vi "Object Factory.vi"(6 "Ring Images In":variant, 8 "error in (no error)":errorcluster, 9 "Panel Origin":T1, 11 "GOject In":refnum<vi>) -> (0 "error out":errorcluster, 1 "Is Visible":bool, 2 "Is Control":bool, 3 "Object Out":refnum<class "Object.lvclass">, 4 "Ring Images Out":variant, 5 "Is Indicator":bool)   [LabVIEW 2015, in "Front Panel Publisher.lvlib" / "Web Front Panel.lvclass"]
doc: "Convert FP refs into \"HTML\" objects"
uses:
  Web Front Panel.lvclass
  Front Panel Objects/Object_class/Object.lvclass
  <vilib>/Utility/miscctls.llb/LVPointTypeDef.ctl
  Front Panel Objects/Object_class/Attributes.ctl
  Front Panel Objects/Object_class/Coordinates.ctl
  Front Panel Objects/Control_class/Attributes.ctl
  Front Panel Objects/Text_class/Text.lvclass
  Front Panel Objects/Boolean_class/Attributes.ctl
  Front Panel Objects/Numeric_class/Attributes.ctl
  Front Panel Objects/String_class/Attributes.ctl
  Front Panel Objects/Graph_class/Attributes.ctl
  Front Panel Objects/Select_class/Attributes.ctl
  Front Panel Objects/Progressbar_class/Attributes.ctl
  Front Panel Objects/Text_class/Attributes.ctl
  Front Panel Objects/Control_class/Control.lvclass
  Front Panel Objects/Boolean_class/Boolean.lvclass
  Front Panel Objects/Graph_class/Graph.lvclass
  Front Panel Objects/Numeric_class/Numeric.lvclass
  Front Panel Publisher.lvlib
  Front Panel Objects/String_class/String.lvclass
  Front Panel Objects/Select_class/Select.lvclass
  Front Panel Objects/Progressbar_class/Progressbar.lvclass
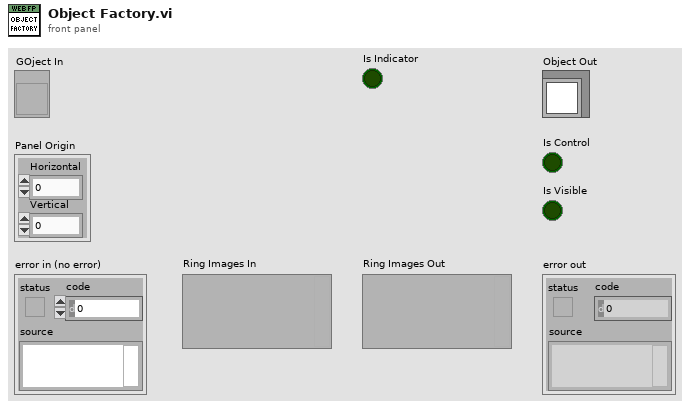
[diagram p1: front panel]
types:
  T1 = typedef "LVPointTypeDef.ctl" = cluster{"Horizontal":i16, "Vertical":i16}
  T2 = typedef "Front Panel Publisher.lvlib/Object.lvclass/Attributes.ctl" = cluster{"UID":i32, "Type":string, "Coordinates":T3, "Reference":refnum<vi>}
  T3 = typedef "Front Panel Publisher.lvlib/Object.lvclass/Coordinates.ctl" = cluster{"Left":i32, "Top":i32, "Height":u32, "Width":u32}
  T4 = typedef "Front Panel Publisher.lvlib/Control.lvclass/Attributes.ctl" = cluster{"Description":string, "Indicator":bool, "Default Value":variant, "Control Index":i32, "Label":refnum<class "Text.lvclass">, "Caption":refnum<class "Text.lvclass">, "Image b64":string, "Use Picture":bool, "Value Only":bool}
  T5 = typedef "Front Panel Publisher.lvlib/Boolean.lvclass/Attributes.ctl" = cluster{"Boolean ref":refnum<vi>, "Switching":bool, "Boolean Strings":string[], "Text":refnum<class "Text.lvclass">, "Images b64":string[]}
  T6 = typedef "Front Panel Publisher.lvlib/Numeric.lvclass/Attributes.ctl" = cluster{"unused":dbl}
  T7 = typedef "Front Panel Publisher.lvlib/String.lvclass/Attributes.ctl" = cluster{"unused":string}
  T8 = typedef "Front Panel Publisher.lvlib/Graph.lvclass/Attributes.ctl" = cluster{"X Label Text":string, "X Format String":string, "Y Label Text":string[], "Y Format String":string[], "Plot Y Axis Selection":enum16{"Y Axis", "Y2 Axis"}[], "Width":u32, "Series JSON Data":string}
  T9 = typedef "Front Panel Publisher.lvlib/Select.lvclass/Attributes.ctl" = cluster{"Ring Image Variable Name":string}
  T10 = typedef "Front Panel Publisher.lvlib/Progressbar.lvclass/Attributes.ctl" = cluster{"Maximum":dbl, "Minimum":dbl}
  T11 = cluster{"Object":T2, "Control":T4, "Boolean":T5, "Numeric":T6, "String":T7, "Graph":T8, "Select":T9, "Progressbar":T10, "Object out":refnum<class "Object.lvclass">, "Label":refnum<class "Text.lvclass">, "Caption":refnum<class "Text.lvclass">, "Is Indicator":bool, "Is Control":bool, "Is Visible":bool, "Ring Images":variant}
  T12 = typedef "Front Panel Publisher.lvlib/Text.lvclass/Attributes.ctl" = cluster{"Text":string, "Font":string, "Font Size":u32, "Visible":bool, "Control Reference":refnum<vi>}
  T13 = typedef "LVRectTypeDef.ctl" = cluster{"Left":i16, "Top":i16, "Right":i16, "Bottom":i16}
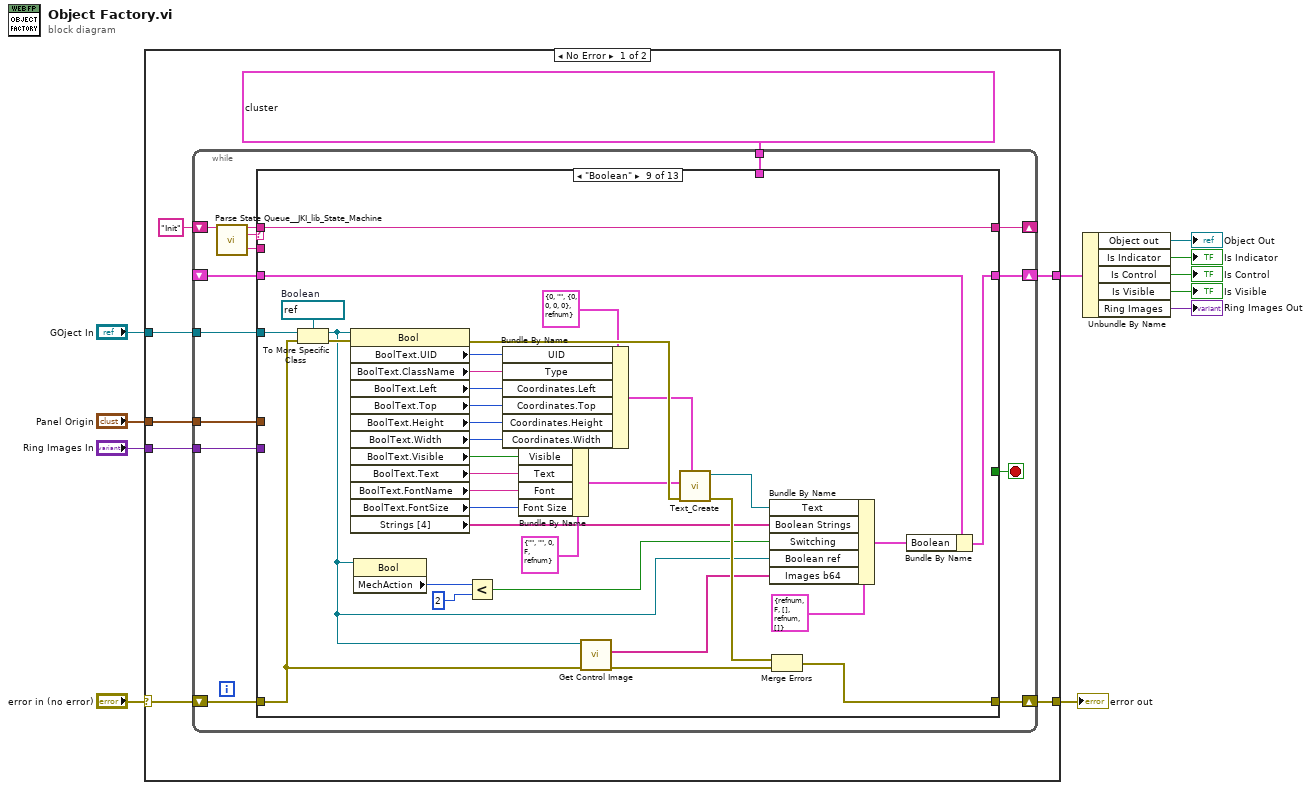
[diagram p0: block diagram]
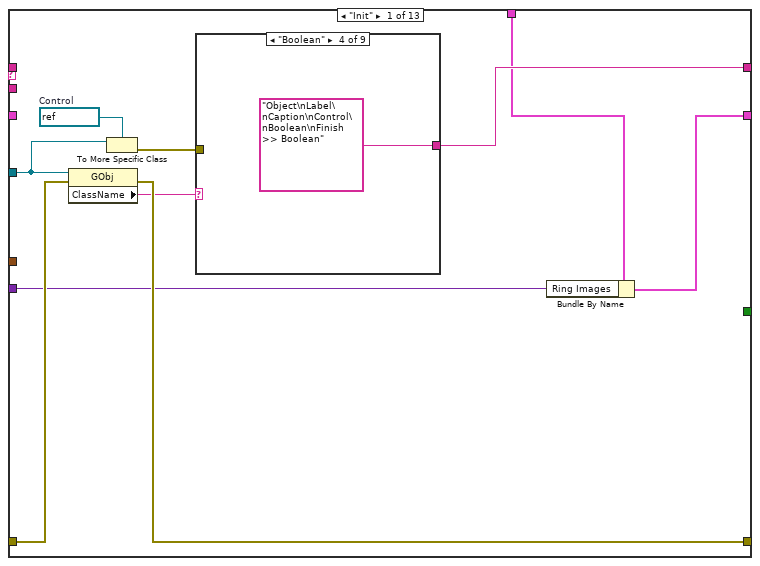
[diagram p2: hidden frame]
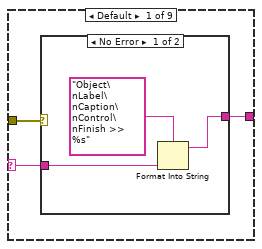
[diagram p3: hidden frame]
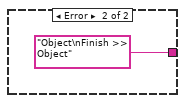
[diagram p4: hidden frame]
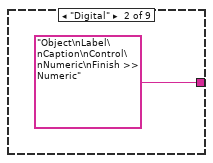
[diagram p5: hidden frame]
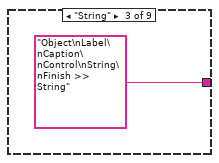
[diagram p6: hidden frame]
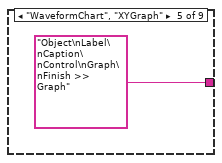
[diagram p7: hidden frame]
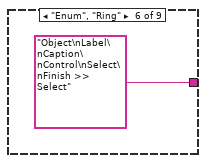
[diagram p8: hidden frame]
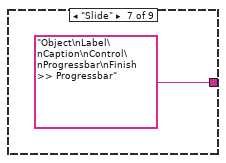
[diagram p9: hidden frame]
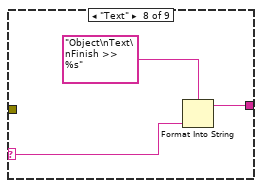
[diagram p10: hidden frame]
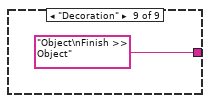
[diagram p11: hidden frame]
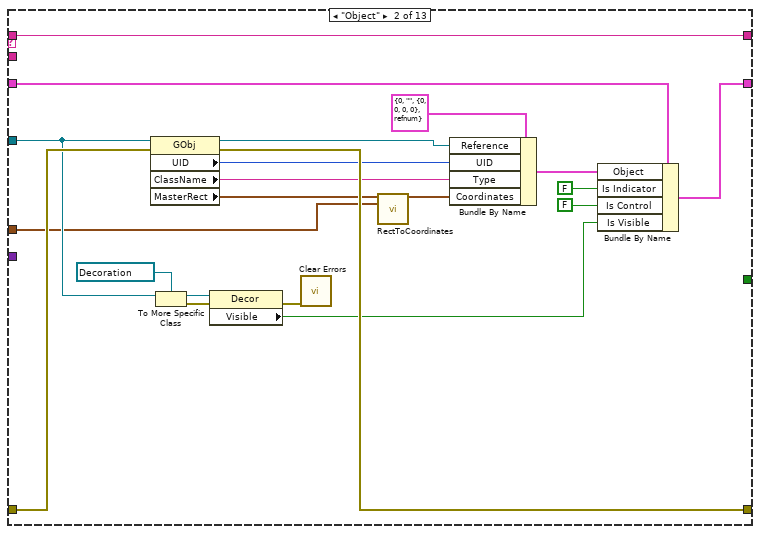
[diagram p12: hidden frame]
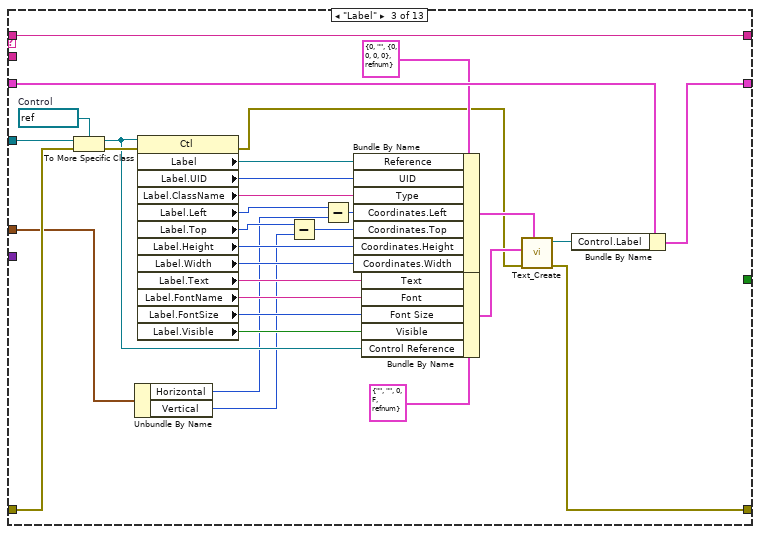
[diagram p13: hidden frame]
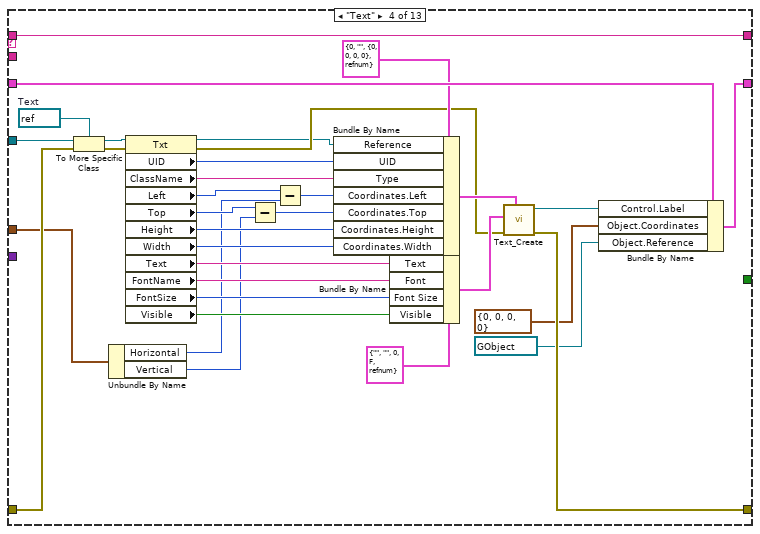
[diagram p14: hidden frame]
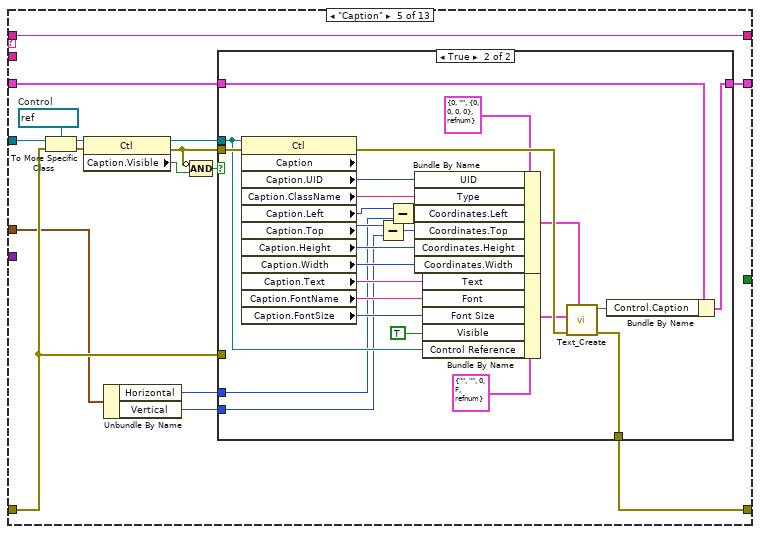
[diagram p15: hidden frame]
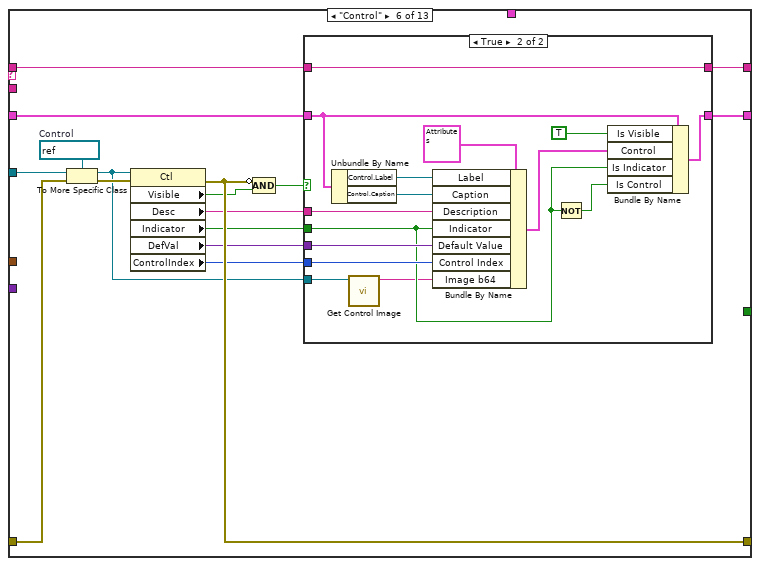
[diagram p17: hidden frame]
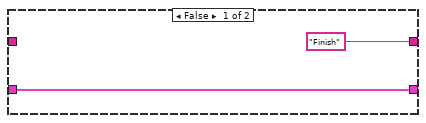
[diagram p18: hidden frame]
diagram:
  n1 = case shown="No Error" "error in (no error)" {
    selector: "error in (no error)" -> [w18 w353]
    tunnel: [w19 w353] -> w10
    tunnel: "GOject In" -> [w17 _]
    tunnel: [w14 _] -> w8
    tunnel: "Ring Images In" -> [w13 _]
    tunnel: "Panel Origin" -> [w12 _]
    frame No Error {
      n2 = while {
        tunnel: w17 -> [w31]
        shift-right: [w22] -> _
        shift-left: "Init" -> [w26]
        shift-right: [w30] -> w14
        shift-left: _ -> [w29]
        shift-right: [w32] -> w19
        shift-left: w18 -> [w33]
        tunnel: T11 {"Object"={"UID"=0, "Type"="", "Coordinates"={"Left"=0, "Top"=0, "Height"=0, "Width"=0}, "Reference"=refnum}, "Control"={"Description"="", "Indicator"=FALSE, "Default Value"=variant, "Control Index"=0, "Label"=refnum, "Caption"=refnum, "Image b64"="", "Use Picture"=FALSE, "Value Only"=FALSE}, "Boolean"={"Boolean ref"=refnum, "Switching"=FALSE, "Boolean Strings"=[], "Text"=refnum, "Images b64"=[]}, "Numeric"={"unused"=0.0}, "String"={"unused"=""}, "Graph"={"X Label Text"="", "X Format String"="", "Y Label Text"=[], "Y Format String"=[], "Plot Y Axis Selection"=[], "Width"=0, "Series JSON Data"=""}, "Select"={"Ring Image Variable Name"=""}, "Progressbar"={"Maximum"=0.0, "Minimum"=0.0}, "Object out"=refnum, "Label"=refnum, "Caption"=refnum, "Is Indicator"=FALSE, "Is Control"=FALSE, "Is Visible"=FALSE, "Ring Images"=variant} -> [w28]
        tunnel: w13 -> [w21]
        tunnel: w12 -> [w20]
        stop <- w27 stop-if-true
        n3 = call <vilib>:"Parse State Queue__JKI_lib_State_Machine.vi"("State Queue"=w26) -> ("Remaining States"=w23:string, "Current State"=w25:string, "Arguments"=w24:string)  [unwired: 12 in]
        n4 = case shown="\"Boolean\"" w25 {
          tunnel: w31 -> [w38 w68 w108 w141 w155 w200 _ _ w259 w267 w272 w285 _]
          tunnel: [w40 w75 w96 w129 w150 w191 w224 w227 w256 w271 w280 w291 ""] -> w22
          tunnel: [w35 w77 w97 w130 w151 w194 w223 w226 w257 w269 w278 w290 w293] -> w30
          tunnel: w29 -> [_ w76 w98 w131 w152 w199 w223 w226 w258 w270 w279 w289 w292]
          tunnel: [w42 w80 w110 w143 w159 w202 w222 w225 w229 w262 w276 w281 w297] -> w32
          tunnel: w33 -> [w43 w81 w111 w144 w158 w203 w222 w225 w230 w263 w273 w282 w297]
          tunnel: w28 -> [w39 _ _ _ _ _ _ _ _ _ _ _ _]
          tunnel: [_ _ _ _ _ _ _ _ _ _ _ _ TRUE] -> w27
          tunnel: w24 -> [_ _ _ _ _ _ _ _ _ _ _ _ w294]
          tunnel: w23 -> [_ w75 w96 w129 w150 w190 w224 w227 w256 w271 w280 w291 _]
          tunnel: w21 -> [w34 _ _ _ _ _ _ _ _ _ w275 _ _]
          tunnel: w20 -> [_ w61 w84 w115 w148 _ _ _ _ _ _ _ _]
          frame "Init" {
            w37 = refnum<vi> refnum  # Control
            n5 = property class="GObj"(reference=w38, error in=w43) -> (error out=w42:errorcluster, "ClassName"=w41:string)  [unwired: 1 out]
            n6 = To More Specific Class(target class=w37, reference=w38) -> (error out=w36:errorcluster)  [unwired: 1 in, 1 out]
            n7 = case shown="\"Boolean\"" w41 {
              selector: w41 -> [w44 _ _ _ _ _ _ w58 _]
              tunnel: [w46 "Object\nLabel\nCaption\nControl\nNumeric\nFinish >> Numeric" "Object\nLabel\nCaption\nControl\nString\nFinish >> String" "Object\nLabel\nCaption\nControl\nBoolean\nFinish >> Boolean" "Object\nLabel\nCaption\nControl\nGraph\nFinish >> Graph" "Object\nLabel\nCaption\nControl\nSelect\nFinish >> Select" "Object\nLabel\nCaption\nControl\nProgressbar\nFinish >> Progressbar" w57 "Object\nFinish >> Object"] -> w40
              tunnel: w36 -> [w45 _ _ _ _ _ _ _ _]
              frame Default {
                n8 = case shown="No Error" w45 {
                  tunnel: [w47 "Object\nFinish >> Object"] -> w46
                  tunnel: w44 -> [w49 _]
                  frame No Error {
                    n9 = Format Into String(format string="Object\nLabel\nCaption\nControl\nFinish >> %s", w49) -> (resulting string=w47:string)  [unwired: 2 in, 1 out]
                  }
                  frame Error {
                  }
                }
              }
              frame "Digital" {
              }
              frame "String" {
              }
              frame "Boolean" {
              }
              frame "WaveformChart", "XYGraph" {
              }
              frame "Enum", "Ring" {
              }
              frame "Slide" {
              }
              frame "Text" {
                n10 = Format Into String(format string="Object\nText\nFinish >> %s", w58) -> (resulting string=w57:string)  [unwired: 2 in, 1 out]
              }
              frame "Decoration" {
              }
            }
            n11 = Bundle By Name(cluster=w39, "Ring Images"=w34) -> (w35:T11)
          }
          frame "Object" {
            n12 = property class="GObj"(reference=w68, error in=w81) -> (reference out=w71:refnum<vi>, error out=w80:errorcluster, "UID"=w78:i32, "ClassName"=w79:string, "MasterRect"=w72:T13)
            n13 = To More Specific Class(target class=refnum<vi> refnum ("GOject"), reference=w68) -> (specific class reference=w67:refnum<vi>, error out=w66:errorcluster)  [unwired: 1 in]
            n14 = property class="Decor"(reference=w67, error in=w66) -> (error out=w65:errorcluster, "Visible"=w64:bool)  [unwired: 1 out]
            n15 = call <vilib>:"Clear Errors.vi"("error in (no error)"=w65) -> ()  [unwired: 5 in, 2 out]
            n16 = call "RectToCoordinates.vi"("Rect"=w72, "Panel Origin"=w61) -> ("Coordinates"=w70:T3)  [unwired: 13 in]
            n17 = Bundle By Name(cluster=T2 {"UID"=0, "Type"="", "Coordinates"={"Left"=0, "Top"=0, "Height"=0, "Width"=0}, "Reference"=refnum} ("Object Attributes"), "Reference"=w71, "UID"=w78, "Type"=w79, "Coordinates"=w70) -> (w73:T2)
            n18 = Bundle By Name(cluster=w76, "Object"=w73, "Is Indicator"=FALSE, "Is Control"=FALSE, "Is Visible"=w64) -> (w77:T11)
          }
          frame "Label" {
            w109 = refnum<vi> refnum  # Control
            n19 = To More Specific Class(target class=w109, reference=w108, error in=w111) -> (specific class reference=w87:refnum<vi>, error out=w112:errorcluster)
            n20 = Unbundle By Name(w84) -> ("Horizontal"=w83:i16, "Vertical"=w82:i16)
            n21 = property class="Ctl"(reference=w87, error in=w112) -> (error out=w90:errorcluster, "Label"=w88:refnum<vi>, "Label.UID"=w107:i32, "Label.ClassName"=w106:string, "Label.Left"=w105:i32, "Label.Top"=w104:i32, "Label.Height"=w103:u32, "Label.Width"=w102:u32, "Label.Text"=w101:string, "Label.FontName"=w100:string, "Label.FontSize"=w99:u32, "Label.Visible"=w89:bool)  [unwired: 1 out]
            n22 = Subtract(x=w104, y=w82) -> (x-y=w85:i32)
            n23 = Subtract(x=w105, y=w83) -> (x-y=w86:i32)
            n24 = Bundle By Name(cluster=T2 {"UID"=0, "Type"="", "Coordinates"={"Left"=0, "Top"=0, "Height"=0, "Width"=0}, "Reference"=refnum} ("Object Attributes"), "Reference"=w88, "UID"=w107, "Type"=w106, "Coordinates.Left"=w86, "Coordinates.Top"=w85, "Coordinates.Height"=w103, "Coordinates.Width"=w102) -> (w93:T2)
            n25 = Bundle By Name(cluster=T12 {"Text"="", "Font"="", "Font Size"=0, "Visible"=FALSE, "Control Reference"=refnum} ("Text Attributes"), "Text"=w101, "Font"=w100, "Font Size"=w99, "Visible"=w89, "Control Reference"=w87) -> (w92:T12)
            n26 = call "Text_Create.vi"("Object Attributes"=w93, "error in (no error)"=w90, "Text Attributes"=w92) -> ("error out"=w110:errorcluster, "Text Out"=w91:refnum<class "Text.lvclass">)  [unwired: 7 in]
            n27 = Bundle By Name(cluster=w98, "Control.Label"=w91) -> (w97:T11)
          }
          frame "Text" {
            w142 = refnum<vi> refnum  # Text
            n28 = To More Specific Class(target class=w142, reference=w141, error in=w144) -> (specific class reference=w121:refnum<vi>, error out=w145:errorcluster)
            n29 = Unbundle By Name(w115) -> ("Horizontal"=w114:i16, "Vertical"=w113:i16)
            n30 = property class="Txt"(reference=w121, error in=w145) -> (reference out=w120:refnum<vi>, error out=w123:errorcluster, "UID"=w140:i32, "ClassName"=w139:string, "Left"=w138:i32, "Top"=w137:i32, "Height"=w136:u32, "Width"=w135:u32, "Text"=w134:string, "FontName"=w133:string, "FontSize"=w132:u32, "Visible"=w122:bool)
            n31 = Subtract(x=w137, y=w113) -> (x-y=w116:i32)
            n32 = Subtract(x=w138, y=w114) -> (x-y=w117:i32)
            n33 = Bundle By Name(cluster=T2 {"UID"=0, "Type"="", "Coordinates"={"Left"=0, "Top"=0, "Height"=0, "Width"=0}, "Reference"=refnum} ("Object Attributes"), "Reference"=w120, "UID"=w140, "Type"=w139, "Coordinates.Left"=w117, "Coordinates.Top"=w116, "Coordinates.Height"=w136, "Coordinates.Width"=w135) -> (w126:T2)
            n34 = Bundle By Name(cluster=T12 {"Text"="", "Font"="", "Font Size"=0, "Visible"=FALSE, "Control Reference"=refnum} ("Text Attributes"), "Text"=w134, "Font"=w133, "Font Size"=w132, "Visible"=w122) -> (w125:T12)
            n35 = call "Text_Create.vi"("Object Attributes"=w126, "error in (no error)"=w123, "Text Attributes"=w125) -> ("error out"=w143:errorcluster, "Text Out"=w124:refnum<class "Text.lvclass">)  [unwired: 7 in]
            n36 = Bundle By Name(cluster=w131, "Control.Label"=w124, "Object.Coordinates"=T3 {"Left"=0, "Top"=0, "Height"=0, "Width"=0}, "Object.Reference"=refnum<vi> refnum) -> (w130:T11)
          }
          frame "Caption" {
            w157 = refnum<vi> refnum  # Control
            n37 = To More Specific Class(target class=w157, reference=w155, error in=w158) -> (specific class reference=w156:refnum<vi>, error out=w161:errorcluster)
            n38 = property class="Ctl"(reference=w156, error in=w161) -> (reference out=w149:refnum<vi>, error out=w160:errorcluster, "Caption.Visible"=w154:bool)
            n39 = Unbundle By Name(w148) -> ("Horizontal"=w147:i16, "Vertical"=w146:i16)
            n40 = Compound Arithmetic op=AND(invert w160, w154) -> (w153:bool)
            n41 = case shown="True" w153 {
              tunnel: w152 -> [w162 w181]
              tunnel: [w162 w180] -> w151
              tunnel: w149 -> [_ w168]
              tunnel: w160 -> [_ w188]
              tunnel: [w163 w186] -> w159
              tunnel: w158 -> [w163 _]
              tunnel: w147 -> [_ w165]
              tunnel: w146 -> [_ w164]
              frame False {
              }
              frame True {
                n42 = property class="Ctl" props=["Caption", "Caption", "UID", "Caption", "ClassName", "Caption", "Left", "Caption", "Top", "Caption", "Height", "Caption", "Width", "Caption", "Text", "Caption", "FontName", "Caption", "FontSize"](reference=w168, error in=w188) -> (error out=w187:errorcluster, "Caption.UID"=w178:i32, "Caption.ClassName"=w177:string, "Caption.Left"=w176:i32, "Caption.Top"=w175:i32, "Caption.Height"=w174:u32, "Caption.Width"=w173:u32, "Caption.Text"=w172:string, "Caption.FontName"=w171:string, "Caption.FontSize"=w170:u32)  [unwired: 2 out]
                n43 = Subtract(x=w175, y=w164) -> (x-y=w166:i32)
                n44 = Subtract(x=w176, y=w165) -> (x-y=w167:i32)
                n45 = Bundle By Name(cluster=T2 {"UID"=0, "Type"="", "Coordinates"={"Left"=0, "Top"=0, "Height"=0, "Width"=0}, "Reference"=refnum} ("Object Attributes"), "UID"=w178, "Type"=w177, "Coordinates.Left"=w167, "Coordinates.Top"=w166, "Coordinates.Height"=w174, "Coordinates.Width"=w173) -> (w183:T2)
                n46 = Bundle By Name(cluster=T12 {"Text"="", "Font"="", "Font Size"=0, "Visible"=FALSE, "Control Reference"=refnum} ("Text Attributes"), "Text"=w172, "Font"=w171, "Font Size"=w170, "Visible"=TRUE, "Control Reference"=w168) -> (w182:T12)
                n47 = call "Text_Create.vi"("Object Attributes"=w183, "error in (no error)"=w187, "Text Attributes"=w182) -> ("error out"=w186:errorcluster, "Text Out"=w179:refnum<class "Text.lvclass">)  [unwired: 7 in]
                n48 = Bundle By Name(cluster=w181, "Control.Caption"=w179) -> (w180:T11)
              }
            }
          }
          frame "Control" {
            w201 = refnum<vi> refnum  # Control
            n49 = To More Specific Class(target class=w201, reference=w200, error in=w203) -> (specific class reference=w189:refnum<vi>, error out=w204:errorcluster)
            n50 = property class="Ctl"(reference=w189, error in=w204) -> (error out=w202:errorcluster, "Visible"=w192:bool, "Desc"=w198:string, "Indicator"=w197:bool, "DefVal"=w196:variant, "ControlIndex"=w195:i32)  [unwired: 1 out]
            n51 = Compound Arithmetic op=AND(invert w202, w192) -> (w193:bool)
            n52 = case shown="True" w193 {
              tunnel: w199 -> [w206 w215]
              tunnel: w198 -> [_ w221]
              tunnel: w197 -> [_ w211]
              tunnel: w196 -> [_ w220]
              tunnel: w195 -> [_ w219]
              tunnel: [w206 w208] -> w194
              tunnel: ["Finish" w216] -> w191
              tunnel: w190 -> [_ w216]
              tunnel: w189 -> [_ w209]
              frame False {
              }
              frame True {
                n53 = Unbundle By Name(w215) -> ("Control.Label"=w214:refnum<class "Text.lvclass">, "Control.Caption"=w213:refnum<class "Text.lvclass">)
                n54 = call "Get Control Image.vi"("Control ref"=w209) -> ("base64 encoded <img>"=w207:string)  [unwired: 8 in, 2 out]
                n55 = Bundle By Name(cluster=T4 {"Description"="", "Indicator"=FALSE, "Default Value"=variant, "Control Index"=0, "Label"=refnum, "Caption"=refnum, "Image b64"="", "Use Picture"=FALSE, "Value Only"=FALSE} ("Control Attributes"), "Label"=w214, "Caption"=w213, "Description"=w221, "Indicator"=w211, "Default Value"=w220, "Control Index"=w219, "Image b64"=w207) -> (w217:T4)
                n56 = Not(x=w211) -> (.not. x?=w210:bool)
                n57 = Bundle By Name(cluster=w215, "Is Visible"=TRUE, "Control"=w217, "Is Indicator"=w211, "Is Control"=w210) -> (w208:T11)
              }
            }
          }
          frame "Numeric" {
            # "All properties are queried at run time"
          }
          frame "String" {
            # "All properties are queried at run time"
          }
          frame "Boolean" {
            w260 = refnum<vi> refnum  # Boolean
            n58 = To More Specific Class(target class=w260, reference=w259, error in=w230) -> (specific class reference=w232:refnum<vi>, error out=w234:errorcluster)
            n59 = property class="Bool"(reference=w232, error in=w234) -> (error out=w255:errorcluster, "BoolText.UID"=w245:i32, "BoolText.ClassName"=w244:string, "BoolText.Left"=w243:i32, "BoolText.Top"=w242:i32, "BoolText.Height"=w241:u32, "BoolText.Width"=w240:u32, "BoolText.Visible"=w235:bool, "BoolText.Text"=w239:string, "BoolText.FontName"=w238:string, "BoolText.FontSize"=w237:u32, "Strings [4]"=w236:string[])  [unwired: 1 out]
            n60 = property class="Bool"(reference=w232) -> ("MechAction"=w233:u32)  [unwired: 1 in, 2 out]
            n61 = Less?(x=w233, y=u32 2) -> (x < y?=w246:bool)
            n62 = Bundle By Name(cluster=T2 {"UID"=0, "Type"="", "Coordinates"={"Left"=0, "Top"=0, "Height"=0, "Width"=0}, "Reference"=refnum} ("Object Attributes"), "UID"=w245, "Type"=w244, "Coordinates.Left"=w243, "Coordinates.Top"=w242, "Coordinates.Height"=w241, "Coordinates.Width"=w240) -> (w250:T2)
            n63 = Bundle By Name(cluster=T12 {"Text"="", "Font"="", "Font Size"=0, "Visible"=FALSE, "Control Reference"=refnum} ("Text Attributes"), "Visible"=w235, "Text"=w239, "Font"=w238, "Font Size"=w237) -> (w249:T12)
            n64 = call "Get Control Image.vi"("error in (no error)"=w230, "Control ref"=w232) -> ("error out"=w228:errorcluster, "All base64 Images"=w231:string[])  [unwired: 7 in, 1 out]
            n65 = call "Text_Create.vi"("Object Attributes"=w250, "error in (no error)"=w255, "Text Attributes"=w249) -> ("error out"=w261:errorcluster, "Text Out"=w248:refnum<class "Text.lvclass">)  [unwired: 7 in]
            n66 = Bundle By Name(cluster=T5 {"Boolean ref"=refnum, "Switching"=FALSE, "Boolean Strings"=[], "Text"=refnum, "Images b64"=[]} ("BooleanControl Attributes"), "Text"=w248, "Boolean Strings"=w236, "Switching"=w246, "Boolean ref"=w232, "Images b64"=w231) -> (w247:T5)
            n67 = Merge Errors(w261, w228) -> (w229:errorcluster)
            n68 = Bundle By Name(cluster=w258, "Boolean"=w247) -> (w257:T11)
          }
          frame "Graph", Default {
            w268 = refnum<vi> refnum  # XYGraph
            n69 = To More Specific Class(target class=w268, reference=w267, error in=w263) -> (specific class reference=w266:refnum<vi>, error out=w265:errorcluster)
            n70 = property class="XYGraph"(reference=w266, error in=w265) -> (error out=w262:errorcluster, "Width"=w264:u32)  [unwired: 1 out]
            n71 = Bundle By Name(cluster=w270, "Graph.Width"=w264) -> (w269:T11)
          }
          frame "Select" {
            n72 = call "Get JS Variables For Picture Ring.vi"("error in (no error)"=w273, "Ring Images In"=w275, "Ring in"=w272) -> ("error out"=w276:errorcluster, "Ring Images Out"=w274:variant, "Ring Image Variable Name"=w277:string)  [unwired: 6 in]
            n73 = Bundle By Name(cluster=w279, "Select.Ring Image Variable Name"=w277, "Ring Images"=w274) -> (w278:T11)
          }
          frame "Progressbar" {
            w288 = refnum<vi> refnum  # Slide
            n74 = To More Specific Class(target class=w288, reference=w285, error in=w282) -> (specific class reference=w286:refnum<vi>, error out=w287:errorcluster)
            n75 = property class="Slide"(reference=w286, error in=w287) -> (error out=w281:errorcluster, "Scale.Maximum"=w284:dbl, "Scale.Minimum"=w283:dbl)  [unwired: 1 out]
            n76 = Bundle By Name(cluster=w289, "Progressbar.Maximum"=w284, "Progressbar.Minimum"=w283) -> (w290:T11)
          }
          frame "Finish" {
            n77 = case shown="\"Select\"" w294 {
              tunnel: [w299 w305 w310 w313 w321 w327 w333 w339 w345 w350] -> w293
              tunnel: w292 -> [w301 w306 w311 w317 w323 w329 w335 w341 w347 w352]
              frame "Object" {
                n78 = Unbundle By Name(w301) -> ("Object"=w300:T2)
                n79 = call "Object_Create.vi"("Object Attributes"=w300) -> ("Object Out"=w298:refnum<class "Object.lvclass">)  [unwired: 9 in, 1 out]
                n80 = Bundle By Name(cluster=w301, "Object out"=w298) -> (w299:T11)
              }
              frame "Control" {
                n81 = Unbundle By Name(w306) -> ("Object"=w303:T2, "Control"=w302:T4)
                n82 = call "Control_Create.vi"("Object Attributes"=w303, "Control Attributes"=w302) -> ("Control Out"=w304:refnum<class "Control.lvclass">)  [unwired: 8 in, 1 out]
                n83 = Bundle By Name(cluster=w306, "Object out"=w304) -> (w305:T11)
              }
              frame "Text" {
                n84 = Unbundle By Name(w311) -> ("Object"=w308:T2, "Control"=w307:T4)
                n85 = call "Control_Create.vi"("Object Attributes"=w308, "Control Attributes"=w307) -> ("Control Out"=w309:refnum<class "Control.lvclass">)  [unwired: 8 in, 1 out]
                n86 = Bundle By Name(cluster=w311, "Object out"=w309) -> (w310:T11)
              }
              frame "Boolean" {
                n87 = Unbundle By Name(w317) -> ("Object"=w316:T2, "Control"=w315:T4, "Boolean"=w314:T5)
                n88 = call "Boolean_Create.vi"("Object Attributes"=w316, "BooleanControl Attributes"=w314, "Control Attributes"=w315) -> ("Boolean Out"=w312:refnum<class "Boolean.lvclass">)  [unwired: 7 in, 1 out]
                n89 = Bundle By Name(cluster=w317, "Object out"=w312) -> (w313:T11)
              }
              frame "Graph" {
                n90 = Unbundle By Name(w323) -> ("Object"=w319:T2, "Control"=w322:T4, "Graph"=w318:T8)
                n91 = call "Graph_Create.vi"("Object Attributes"=w319, "Graph Attributes"=w318, "Control Attributes"=w322) -> ("Graph Out"=w320:refnum<class "Graph.lvclass">)  [unwired: 7 in, 1 out]
                n92 = Bundle By Name(cluster=w323, "Object out"=w320) -> (w321:T11)
              }
              frame "Numeric" {
                n93 = Unbundle By Name(w329) -> ("Object"=w325:T2, "Control"=w328:T4, "Numeric"=w324:T6)
                n94 = call "Numeric_Create.vi"("Object Attributes"=w325, "Graph Attributes"=w324, "Control Attributes"=w328) -> ("Numeric Out"=w326:refnum<class "Numeric.lvclass">)  [unwired: 7 in, 1 out]
                n95 = Bundle By Name(cluster=w329, "Object out"=w326) -> (w327:T11)
              }
              frame "String" {
                n96 = Unbundle By Name(w335) -> ("Object"=w331:T2, "Control"=w334:T4, "String"=w330:T7)
                n97 = call "String_Create.vi"("Object Attributes"=w331, "String Attributes"=w330, "Control Attributes"=w334) -> ("String Out"=w332:refnum<class "String.lvclass">)  [unwired: 7 in, 1 out]
                n98 = Bundle By Name(cluster=w335, "Object out"=w332) -> (w333:T11)
              }
              frame "Select" {
                n99 = Unbundle By Name(w341) -> ("Object"=w337:T2, "Control"=w340:T4, "Select"=w336:T9)
                n100 = call "Select_Create.vi"("Object Attributes"=w337, "Select Attributes"=w336, "Control Attributes"=w340) -> ("Select Out"=w338:refnum<class "Select.lvclass">)  [unwired: 7 in, 1 out]
                n101 = Bundle By Name(cluster=w341, "Object out"=w338) -> (w339:T11)
              }
              frame "Progressbar" {
                n102 = Unbundle By Name(w347) -> ("Object"=w343:T2, "Control"=w346:T4, "Progressbar"=w342:T10)
                n103 = call "Progressbar_Create.vi"("Object Attributes"=w343, "Progressbar Attributes"=w342, "Control Attributes"=w346) -> ("Progress Out"=w344:refnum<class "Progressbar.lvclass">)  [unwired: 7 in, 1 out]
                n104 = Bundle By Name(cluster=w347, "Object out"=w344) -> (w345:T11)
              }
              frame Default {
                n105 = Unbundle By Name(w352) -> ("Object"=w348:T2, "Control"=w351:T4)
                n106 = call "Control_Create.vi"("Object Attributes"=w348, "Control Attributes"=w351) -> ("Control Out"=w349:refnum<class "Control.lvclass">)  [unwired: 8 in, 1 out]
                n107 = Bundle By Name(cluster=w352, "Object out"=w349) -> (w350:T11)
              }
            }
          }
        }
      }
    }
    frame Error {
    }
  }
  "error out" <- w10
  n108 = Unbundle By Name(w8) -> ("Object out"=→"Object Out":refnum<class "Object.lvclass">, "Is Indicator"=→"Is Indicator":bool, "Is Control"=→"Is Control":bool, "Is Visible"=→"Is Visible":bool, "Ring Images"=→"Ring Images Out":variant)
